vi "VI in Ursprung setzen Hilfs VI.vi"(11 "VI Referenz":refnum<vi>) -> ()   [LabVIEW 2020, in "allgemeine Sub-VIs.lvlib"]
uses:
  allgemeine Sub-VIs.lvlib
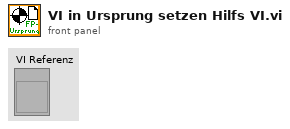
[diagram p1: front panel]
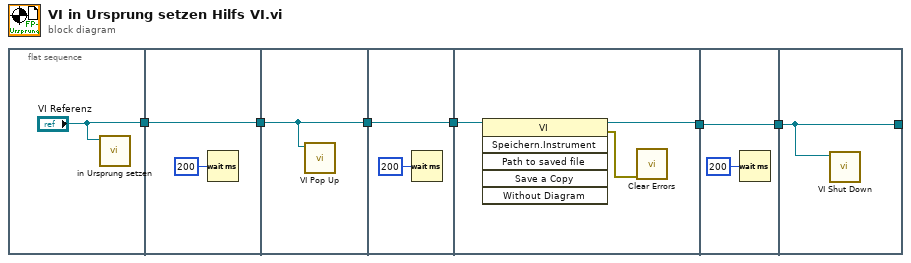
[diagram p0: block diagram]
diagram:
  n1 = flat-sequence {
    tunnel: ["VI Referenz"] -> w6
    tunnel: w6 -> [w9]
    tunnel: [w9] -> w5
    tunnel: w5 -> [w10]
    tunnel: [w10] -> w4
    tunnel: w4 -> [w12]
    tunnel: [w12] -> w3
    tunnel: w3 -> [w15]
    tunnel: [w14] -> w2
    tunnel: w2 -> [w17]
    tunnel: [w17] -> w1
    tunnel: [w18] -> _
    tunnel: w1 -> [w18]
    frame #0 {
      n2 = call "in Ursprung setzen.vi"("VI Referenz"="VI Referenz") -> ()  [unwired: 10 in, 1 out]
    }
    frame #1 {
      n3 = Wait (ms)(milliseconds to wait=u32 200 ("Zu wartende ms")) -> ()  [unwired: 1 out]
    }
    frame #2 {
      n4 = call "VI Pop Up.vi"("VI Referenz"=w10) -> ()  [unwired: 10 in, 1 out]
    }
    frame #3 {
      n5 = Wait (ms)(milliseconds to wait=u32 200 ("Zu wartende ms")) -> ()  [unwired: 1 out]
    }
    frame #4 {
      n6 = invoke class="VI" method="Speichern.Instrument"(reference=w15) -> (reference out=w14:refnum<vi>, error out=w13:errorcluster)  [unwired: 5 in, 4 out]
      n7 = call <vilib>:"Clear Errors.vi"("error in (no error)"=w13) -> ()  [unwired: 5 in, 2 out]
    }
    frame #5 {
      n8 = Wait (ms)(milliseconds to wait=u32 200 ("Zu wartende ms")) -> ()  [unwired: 1 out]
    }
    frame #6 {
      n9 = call "VI Shut Down.vi"("VI Referenz"=w18) -> ()  [unwired: 11 in]
    }
  }
